vi "Homing.vi"(8 "Fehler (Eingang, kein Fehler)":errorcluster) -> (0 "error out":errorcluster)   [LabVIEW 2014]
uses:
  <vilib>/CANopenLib/CANOPEN.llb/CANopen SDO Create.vi
  <vilib>/CANopenLib/CANOPEN.llb/CANopen SDO Read [U32].vi
  <vilib>/CANopenLib/CANOPEN.llb/CANopen SDO Close.vi
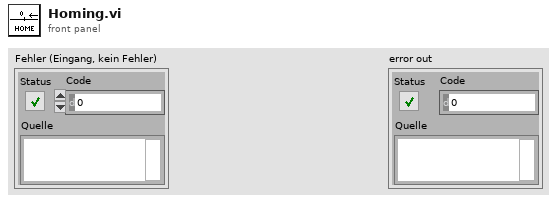
[diagram p1: front panel]
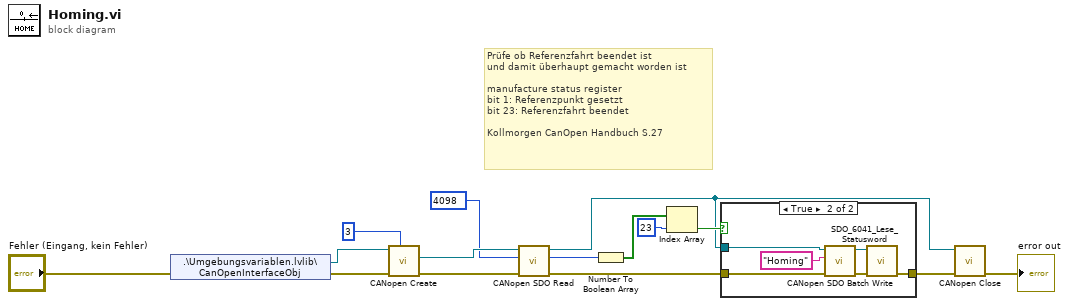
[diagram p0: block diagram]
diagram:
  # "Prüfe ob Referenzfahrt beendet ist\nund damit überhaupt gemacht worden ist \n\nmanufacture status register\nbit 1: Referenzpunkt gesetzt\nbit 23: Referenzfahrt beendet\n\nKollmorgen CanOpen Handbuch S.27"
  n1 = shared-variable ".\\Umgebungsvariablen.lvlib\\CanOpenInterfaceObj"(error in="Fehler (Eingang, kein Fehler)") -> (w15:refnum<k20>, error out=w13:errorcluster)
  n2 = call-poly <vilib>:"CANopen Create.vi"("node-ID"=u8 3, "error in (no error)"=w13, "interface object in"=w15) -> ("error out"=w3:errorcluster, "SDO object out"=w6:refnum<k20>)  [unwired: 6 in, 1 out]
  n3 = call-poly <vilib>:"CANopen SDO Read.vi"("error in (no error)"=w3, "object index"=u16 4098, "SDO object in"=w6) -> ("error out"=w4:errorcluster, "U32 data"=w1:u32, "SDO object out"=w5:refnum<k20>)  [unwired: 5 in, 1 out]
  n4 = Number To Boolean Array(number=w1) -> (Boolean array=w11:bool[])
  n5 = Index Array(array=w11, index=23 ("Index")) -> (element=w9:bool)
  n6 = case shown="True" w9 {
    tunnel: w5 -> [_ w20]
    tunnel: w4 -> [w16 w21]
    tunnel: [w16 w18] -> w8
    frame False {
    }
    frame True {
      n7 = call <vilib>:"CANopen SDO Batch Write.vi"("error in (no error)"=w21, "batch SDO name"="Homing", "SDO object in"=w20) -> ("error out"=w19:errorcluster, "SDO object out"=w17:refnum<k20>)  [unwired: 6 in, 1 out]
      n8 = call "SDO_6041_Lese_Statusword.vi"("error in (no error)"=w19, "SDO object in"=w17) -> ("error out"=w18:errorcluster)  [unwired: 6 in, 3 out]
    }
  }
  n9 = call-poly <vilib>:"CANopen Close.vi"("error in (no error)"=w8, "SDO object in"=w5) -> ("error out"=→"error out":errorcluster)  [unwired: 9 in]
